vi "rising_edge_detection.vi"(10 "input_signal":bool) -> (2 "rising_signal":bool)   [LabVIEW 2020]
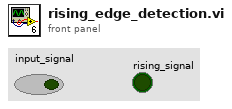
[diagram p1: front panel]
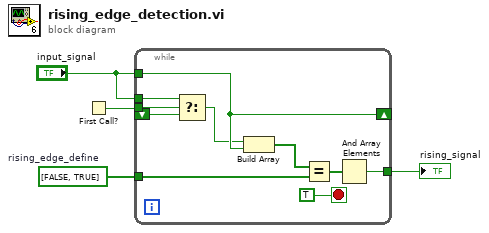
[diagram p0: block diagram]
diagram:
  w3 = bool[] [FALSE, TRUE]  # rising_edge_define
  n1 = First Call?() -> (First Call?: T/F=w2:bool)
  n2 = while {
    shift-right: [w7] -> _
    shift-left: _ -> [w6]
    tunnel: w2 -> [w14]
    tunnel: w3 -> [w12]
    tunnel: [w9] -> w4
    tunnel: "input_signal" -> [w8]
    tunnel: "input_signal" -> [w7]
    stop <- TRUE stop-if-true
    n3 = Select(t=w8, s=w14, f=w6) -> (s? t:f=w5:bool)
    n4 = Build Array(w5, w7) -> (w13:bool[])
    n5 = Equal?(x=w13, y=w12) -> (x = y?=w11:bool[])
    n6 = And Array Elements(Boolean array=w11) -> (logical AND=w9:bool)
  }
  "rising_signal" <- w4
